vi "Network Read.vi"(8 "error in (no error)":errorcluster, 9 "Status_Cluster_in":T1={"simTime"=0.0, "simFrame"=0.0, "Connection Status"=enum."Disconnected", "Connection Command"=enum."Disconnect", "Last Error"=0, "Case selection"=enum."Connecting"}, 10 "RDB References in":T7 {"RDB Send Reference"."RDB Data"."payload" format="%x"; "RDB Send Reference"."RDB Data"."timestamp" format="%<%.7X\n%x>T"; "RDB Send Reference"."RDB Data"."type" items=["FlexRay Data"=32, "FlexRay Null"=33, "FlexRay Symbol"=34, "Log Trigger"=225, "Start Trigger"=226]; "RDB Send Reference"."RDB Data"."cycle count" max=63 step=1; "RDB Receive Reference"."RDB Data"."payload" format="%x"; "RDB Receive Reference"."RDB Data"."timestamp" format="%<%.7X\n%x>T"; "RDB Receive Reference"."RDB Data"."type" items=["FlexRay Data"=32, "FlexRay Null"=33, "FlexRay Symbol"=34, "Log Trigger"=225, "Start Trigger"=226]; "RDB Receive Reference"."RDB Data"."cycle count" max=63 step=1}, 11 "Settings":T4={"UDP Receiver"=refnum, "UDP Sender"=refnum, "Valid Packet"=FALSE, "TCP"=refnum, "Network Settings"={"IP adress"="127.0.0.1", "RDB"={"Protocol"=enum."UDP", "Tx Port"=48270, "Rx Port"=10, "Buffer Size"=204800, "Timeout"=10}, "SCP"={"Protocol"=enum."TCP", "Tx Port"=48191, "Rx Port"=48191, "Buffer Size"=204800, "Timeout"=10}}, "vclient"=path ""}) -> (0 "error out":errorcluster, 1 "Status_Cluster_out":T1={"simTime"=0.0, "simFrame"=0.0, "Connection Status"=enum."Disconnected", "Connection Command"=enum."Disconnect", "Last Error"=0, "Case selection"=enum."Connecting"}, 2 "RDB References out":T7 {"RDB Send Reference"."RDB Data"."payload" format="%x"; "RDB Send Reference"."RDB Data"."timestamp" format="%<%.7X\n%x>T"; "RDB Send Reference"."RDB Data"."type" items=["FlexRay Data"=32, "FlexRay Null"=33, "FlexRay Symbol"=34, "Log Trigger"=225, "Start Trigger"=226]; "RDB Send Reference"."RDB Data"."cycle count" max=63 step=1; "RDB Receive Reference"."RDB Data"."payload" format="%x"; "RDB Receive Reference"."RDB Data"."timestamp" format="%<%.7X\n%x>T"; "RDB Receive Reference"."RDB Data"."type" items=["FlexRay Data"=32, "FlexRay Null"=33, "FlexRay Symbol"=34, "Log Trigger"=225, "Start Trigger"=226]; "RDB Receive Reference"."RDB Data"."cycle count" max=63 step=1}, 3 "Settings":T4={"UDP Receiver"=refnum, "UDP Sender"=refnum, "Valid Packet"=FALSE, "TCP"=refnum, "Network Settings"={"IP adress"="127.0.0.1", "RDB"={"Protocol"=enum."UDP", "Tx Port"=48270, "Rx Port"=10, "Buffer Size"=204800, "Timeout"=10}, "SCP"={"Protocol"=enum."TCP", "Tx Port"=48191, "Rx Port"=48191, "Buffer Size"=204800, "Timeout"=10}}, "vclient"=path ""}, 4 "Packet Size":i32, 5 "RDB Receive Reference.RDB Signals":dbl[](array[numeric]))   [LabVIEW 2023, in "Vires VTD Engine.lvlib"]
uses:
  Vires VTD Engine.lvlib
  RDB/RDB References.ctl
  RDB/RDB Reference.ctl
  <vilib>/xnet/xnet.llb/XNET Frame FlexRay.ctl
  <vilib>/xnet/xnet.llb/XNET Frame Type FlexRay.ctl
  Type/Settings.ctl
  Shared/Network Settings.ctl
  Shared/Protocol.ctl
  Type/Status_Cluster.ctl
  Type/ConnectionStatus.ctl
  Type/CaseSelection.ctl
  RDB/RDB.lvlib
  Utility/Debug_Logger/LoggingProber.lvlib
  Shared/Vires VTD Shared.lvlib
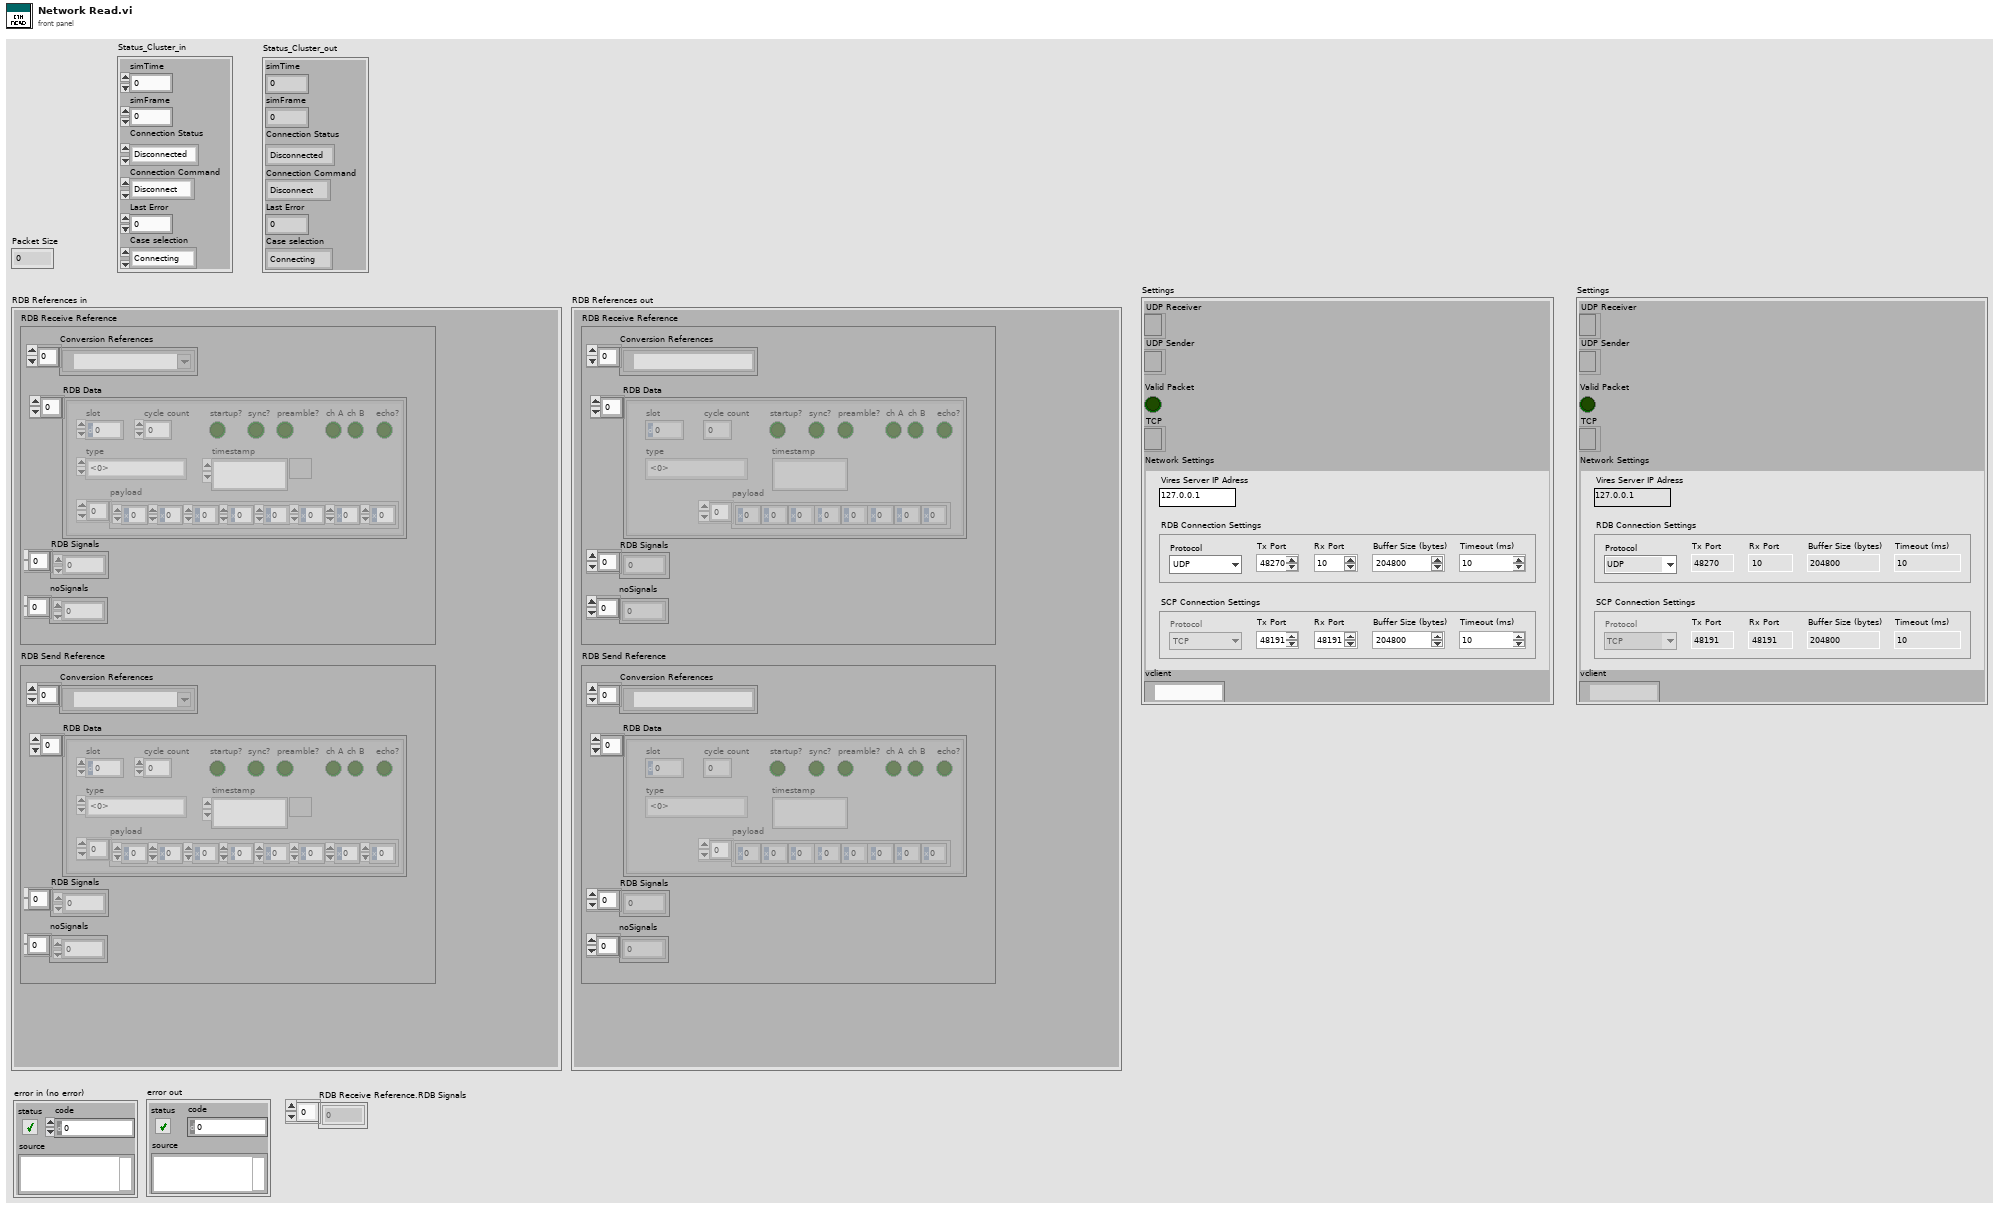
[diagram p1: front panel]
types:
  T1 = typedef "Vires VTD Engine.lvlib/Status_Cluster.ctl" = cluster{"simTime":dbl, "simFrame":dbl, "Connection Status":T2, "Connection Command":enum16{"Disconnect", "Connect"}, "Last Error":i32, "Case selection":T3}
  T2 = typedef "Vires VTD Engine.lvlib/ConnectionStatus.ctl" = enum16{"Disconnected", "Connected"}
  T3 = typedef "Vires VTD Engine.lvlib/CaseSelection.ctl" = enum32{"Idle", "Connecting", "Disconnecting", "Read/Write"}
  T4 = typedef "Vires VTD Engine.lvlib/Settings.ctl" = cluster{"UDP Receiver":refnum<k16>, "UDP Sender":refnum<k16>, "Valid Packet":bool, "TCP":refnum<k5>, "Network Settings":T5, "vclient":path}
  T5 = typedef "Vires VTD Shared.lvlib/Network Settings.ctl" = cluster{"IP adress":string, "RDB":cluster{"Protocol":T6, "Tx Port":u16, "Rx Port":u16, "Buffer Size":i32, "Timeout":u16}, "SCP":cluster{"Protocol":T6, "Tx Port":u16, "Rx Port":u16, "Buffer Size":i32, "Timeout":u16}}
  T6 = typedef "Vires VTD Shared.lvlib/Protocol.ctl" = enum16{"UDP", "TCP"}
  T7 = typedef "RDB.lvlib/RDB References.ctl" = cluster{"RDB Receive Reference":T8, "RDB Send Reference":T8}
  T8 = typedef "RDB.lvlib/RDB Reference.ctl" = cluster{"Conversion References":refnum<k21>[], "RDB Data":T9[], "RDB Signals":dbl[], "noSignals":i32[]}
  T9 = typedef "XNET Frame FlexRay.ctl" = cluster{"timestamp":timestamp, "payload":u8[], "slot":u16, "type":T10, "cycle count":u8, "startup?":bool, "sync?":bool, "preamble?":bool, "ch A":bool, "ch B":bool, "echo?":bool}
  T10 = typedef "XNET Frame Type FlexRay.ctl" = u8
  T11 = enum16{"Standard", "Buffered", "CRLF", "Immediate"}
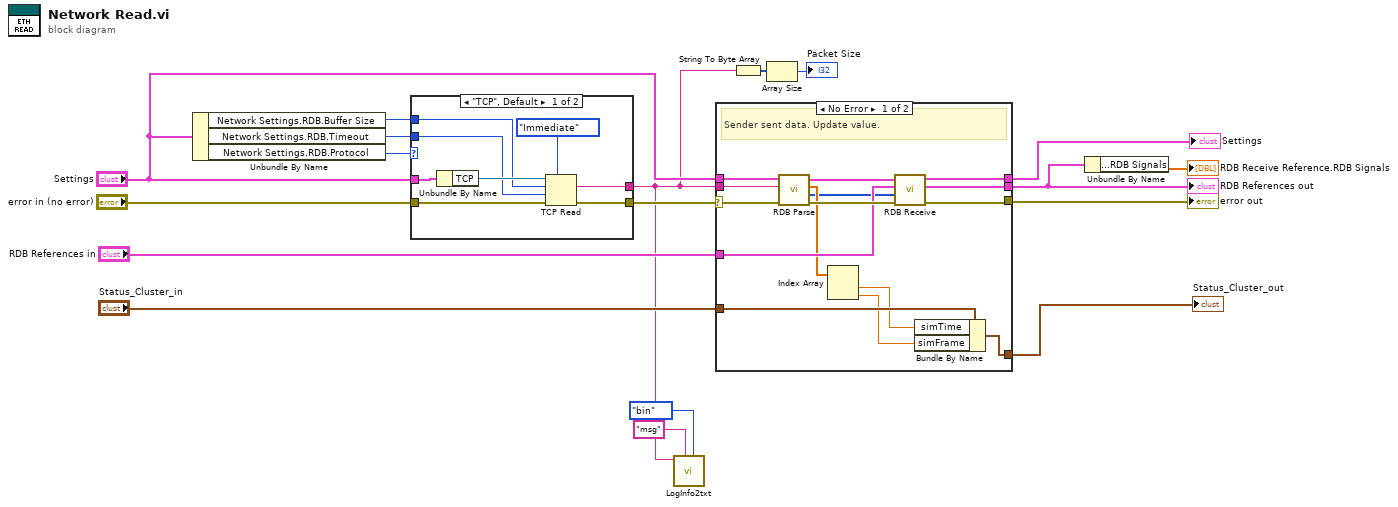
[diagram p0: block diagram]
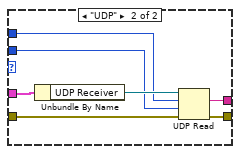
[diagram p2: hidden frame]
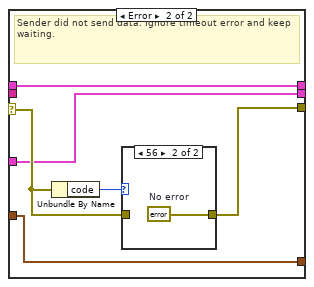
[diagram p3: hidden frame]
diagram:
  n1 = Unbundle By Name("Settings") -> ("Network Settings.RDB.Buffer Size"=w7:i32, "Network Settings.RDB.Timeout"=w8:u16, "Network Settings.RDB.Protocol"=w9:T6)
  n2 = case shown="\"TCP\", Default" w9 {
    tunnel: "error in (no error)" -> [w25 w33]
    tunnel: [w24 w32] -> w17
    tunnel: "Settings" -> [w26 w30]
    tunnel: [w23 w29] -> w3
    tunnel: w7 -> [w19 w28]
    tunnel: w8 -> [w20 w27]
    frame "TCP", Default {
      n3 = Unbundle By Name(w26) -> ("TCP"=w22:refnum<k5>)
      n4 = TCP Read(connection ID=w22, bytes to read=w19, error in (no error)=w25, 7:T11."Immediate" ("mode (standard)"), 9:w20) -> (data out=w23:string, error out=w24:errorcluster)  [unwired: 1 out]
    }
    frame "UDP" {
      n5 = Unbundle By Name(w30) -> ("UDP Receiver"=w31:refnum<k16>)
      n6 = UDP Read(connection ID=w31, max size (548)=w28, timeout ms (25000)=w27, 8:w33) -> (data out=w29:string, error out=w32:errorcluster)  [unwired: 3 out]
    }
  }
  n7 = call "LogInfo2txt.vi"("type"=enum16{"txt", "bin"}."bin", "File ID"="msg", "text"=w3) -> ()  [unwired: 9 in]
  n8 = case shown="No Error" w17 {
    selector: w17 -> [w48 w53]
    tunnel: [w45 w52] -> w15
    tunnel: "RDB References in" -> [w40 w51]
    tunnel: [w44 w51] -> w14
    tunnel: w3 -> [w46 _]
    tunnel: "Settings" -> [w43 w50]
    tunnel: [w41 w50] -> w10
    tunnel: "Status_Cluster_in" -> [w39 w49]
    tunnel: [w36 w49] -> w4
    frame No Error {
      # "Sender sent data. Update value."
      n9 = call "RDB Parse.vi"("error in (no error)"=w48, "RDB Message"=w46, "Settings"=w43) -> ("error out"=w47:errorcluster, "Contact_Point payload"=w34:u8[], "Status"=w37:dbl[], "Settings"=w42:T4)  [unwired: 5 in]
      n10 = Index Array(array=w37) -> (element #1=w38:dbl, element #2=w35:dbl)  [unwired: 2 in]
      n11 = call "RDB Receive.vi"("error in (no error)"=w47, "Payload"=w34, "RDB Reference in"=w40, "Settings"=w42) -> ("error out"=w45:errorcluster, "RDB Reference out"=w44:T7, "Settings"=w41:T4)  [unwired: 5 in]
      n12 = Bundle By Name(cluster=w39, "simTime"=w38, "simFrame"=w35) -> (w36:T1)
    }
    frame Error {
      # "Sender did not send data. Ignore timeout error and keep waiting."
      n13 = Unbundle By Name(w53) -> ("code"=w54:i32)
      n14 = case shown="56" w54 {
        tunnel: w53 -> [w55 _]
        tunnel: [w55 w56] -> w52
        frame Default {
        }
        frame 56 {
          w56 = errorcluster {"status"=FALSE, "code"=0, "source"=""}  # No error
        }
      }
    }
  }
  "RDB References out" <- w14
  "error out" <- w15
  "Settings" <- w10
  "Status_Cluster_out" <- w4
  n15 = String To Byte Array(string=w3) -> (unsigned byte array=w12:u8[])
  n16 = Array Size(array=w12) -> (size(s)=→"Packet Size":i32)
  n17 = Unbundle By Name(w14) -> ("RDB Receive Reference.RDB Signals"=→"RDB Receive Reference.RDB Signals":dbl[])
